vi "8.5.-Momento h2.vi"(1 "n20/n02/n11":dbl[](array[numeric])) -> (0 "M2":dbl)   [LabVIEW 2020]
panel:
  # "Visión Artificial - Momentos Invariantes de Hu\nDiego Cervantes Rodríguez\ndicer0.com"
  # "M2 = ((n20-n02)^2)+((2*n11)^2)"
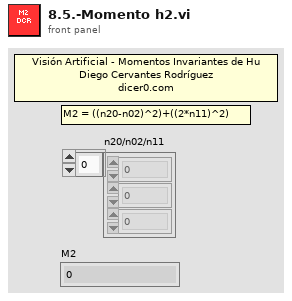
[diagram p1: front panel]
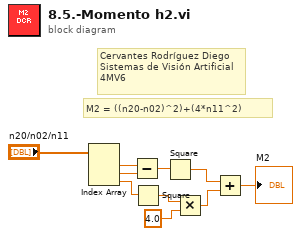
[diagram p0: block diagram]
diagram:
  # "M2 = ((n20-n02)^2)+(4*n11^2)"
  # "Cervantes Rodríguez Diego\nSistemas de Visión Artificial\n4MV6"
  n1 = Index Array "Index Array"(array="n20/n02/n11") -> (element #1=w9:dbl, element #2=w8:dbl, element #3=w6:dbl)  [unwired: 3 in]
  n2 = Subtract(x=w9, y=w8) -> (x-y=w7:dbl)
  n3 = Square(x=w6) -> (x^2=w5:dbl)
  n4 = Square(x=w7) -> (x^2=w3:dbl)
  n5 = Multiply(x=w5, y=4.0) -> (x*y=w2:dbl)
  n6 = Add(x=w3, y=w2) -> (x+y=→"M2":dbl)
